vi "ROI Entry Screen.vi"() -> ()   [LabVIEW 2017]
uses:
  Typedefs/Line draw mode.ctl
  Typedefs/Top level VI states.ctl
  ROI Entry screen/Typedefs/ROI move buttons.ctl
  ROI Entry screen/Typedefs/ROI move mode.ctl
  Typedefs/Offsets cluster.ctl
  Typedefs/ROI management FG states.ctl
  ROI Entry screen/SubVIs/Automatic POI detection/Typedefs/Duplicate POI function enum.ctl
  ROI Entry screen/Typedefs/ROI entry screen ctrl refs cluster.ctl
  Typedefs/Read Write Enum.ctl
  Global Variables/General Globals.vi
  User profiles code/Globals/gl_UsrProfiles globals.vi
  ROI Entry screen/Globals/gl_ROI Entry UI globals.vi
  ROI Entry screen/Typedefs/ROI input mode.ctl
panel:
  out "Current ROI Type":string
  out "AOL Z ind. (um)":dbl caption="Motor Z" format="AOL Z   =  %#_g µm"
  out "# POI":i32 format="%.0f ROI"
  in  "Max Z Proj":bool
  out "ROI":T1
  out "Number of lines left":i32 format="%.0f number of lines left"
  in  "Palette Type":T2(ring)
  out "Zplane ind":i32 caption="Z-Plane" format="Z-Plane %.0f"
  in  "Z-Plane Selector":i32(c297)=7
  out "Image Display":T3(plugin-control)
  out "Motor Z ind. (um)":dbl caption="Motor Z" format="Motor Z = %#_g µm"
  out "# of planes":i32 format="# of Planes = %.0f"
  in  "Intensity slider":cluster{i16, i16}(slide)={0, 4095} caption="Intensity" scale=0.0..4095.0
  in  "Z-stack folder path":path caption="Experiment folder path"
  in  "Channel":enum16{"Green", "Red"}(ring)
  in  "Enable cool-down time":bool caption="Enable stimulus"
  in  "Cool-down time (s)":dbl caption="Cool-down time" min=0.0 max=60.0 step=0.05 format="%#.2f s"
  in  "Enable funct. stimulus":bool caption="Enable stimulus"
  in  "Funct stim.trig.delay (sec)":dbl=0.5 caption="Stimulus trigger delay" min=0.0 max=60.0 step=0.001 format="%#.3fs"
  in  "ROI move mode":T4
  in  "ROI offset arrows":T5
  in  "Trial Length (sec)":dbl=1.0 caption="Trial Length" min=0.05 max=60.0 step=1.0 format="%#.3f s"
  in  "Arb Plane Entry":bool caption="Load\nolder\nPOI"
  in  "Load ROI File":bool caption="Load\nolder\nPOI"
  in  "POI Density":dbl(slide) scale=0.01..1.0
  in  "Auto Generate":bool
  in  "Equal size":bool=TRUE
  in  "Whole plane":bool
  in  "Zoom":dbl=1.0 min=0.001 max=10.0 step=0.1 format="%#.2f x"
  out "Next State":T6=enum."Live Imaging-START"
  in  "Scan dwell time per pixel (us)":dbl=0.1 caption="Scan dwell time\nper pixel (us)" min=0.05 max=20.0 step=0.01 format="%.2f"
  in  "POI dwell time (us)":dbl=4.0 caption="POI dwell time" min=0.05 max=20.0 format="%_3g µs"
  in  "Live Imaging":bool
  in  "Acquisition":bool
  in  "Line Mode":T7=enum."Orthogonal"
  in  "Number of Trials":u16=1 min=1 max=1000 format="%.0f trials"
  in  "Wavelength (nm)":dbl=920.0 caption="Wavelength" min=800.0 max=1080.0 step=1.0 format="%#_g nm"
  in  "Done/Close":bool
  in  "Clear Last":bool
  in  "Clear All":bool
  in  "POISelect Array":cluster{"System Array":dbl[], "Boolean":bool}[](array[cluster])
  in  "Step size (µm)":u8(slide)=1 min=1 max=100 step=1 scale=1.0..30.0
  # "ROI Removal"
  # "ROI Input"
  # "ROI AutoGen"
  # "Min"
  # "Max"
  # "Stimulus trigger delay"
  # "Cool-down time"
  # "ROI Offset"
  # "Settings"
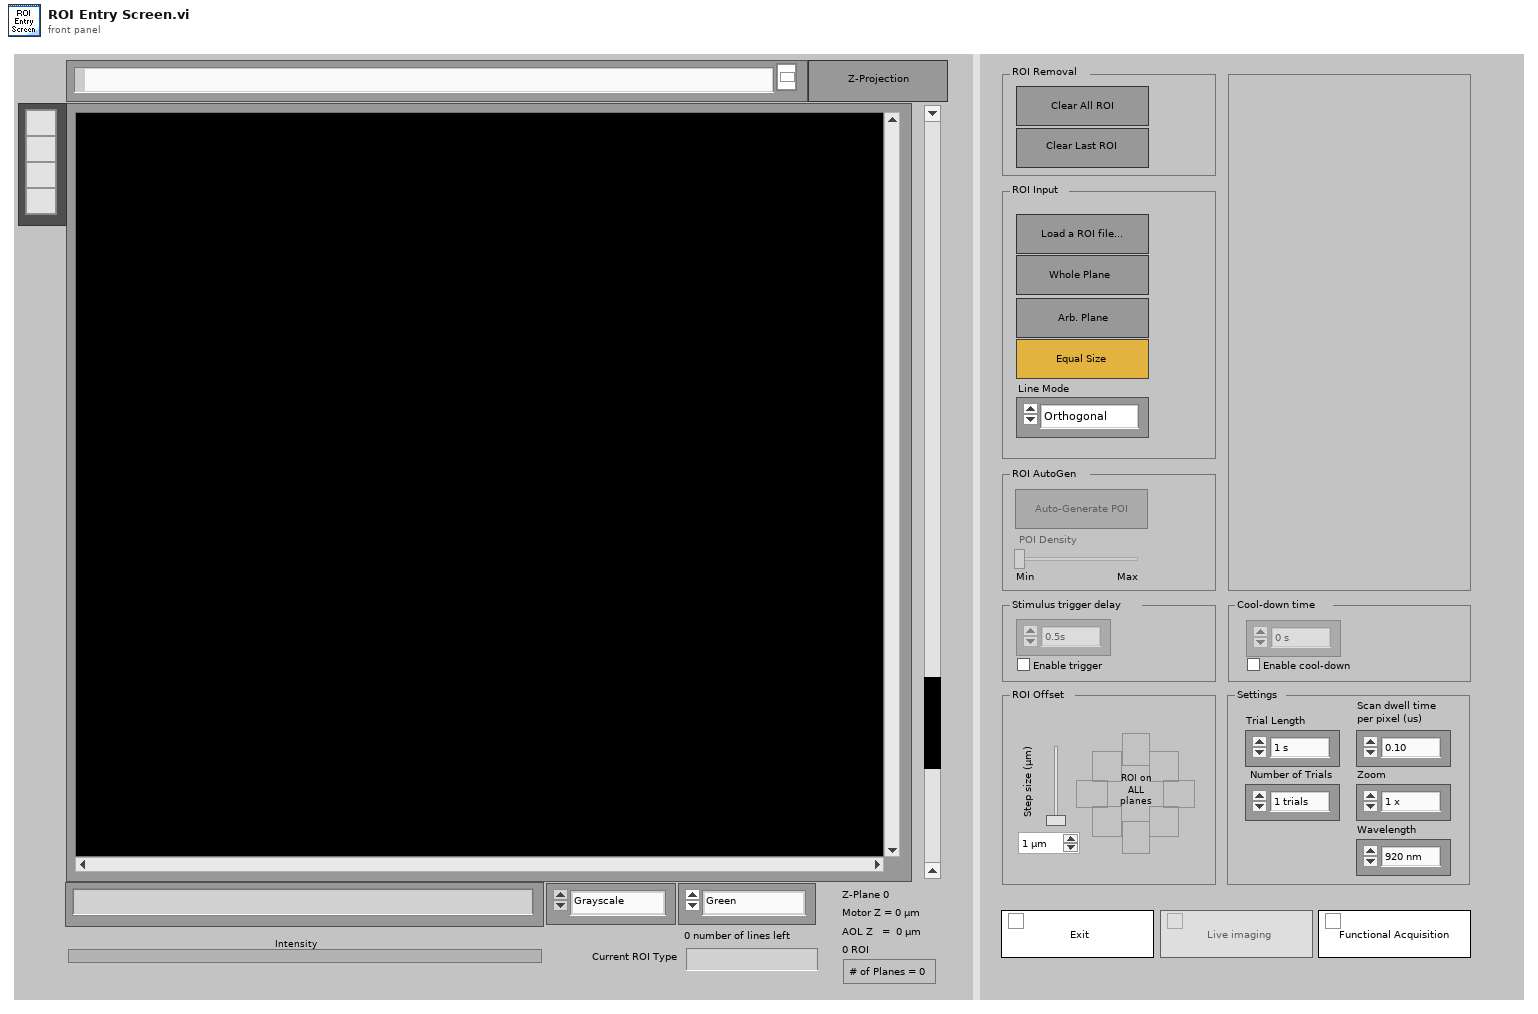
[diagram p1: front panel]
types:
  T1 = cluster{"Global Rectangle":i32[], "Contours":cluster{"Contour Type":u32, "ROI Type":u32, "Points":i32[]}[]}
  T2 = enum16{"Grayscale", "Binary", "Gradient", "Rainbow", "Temperature", "User Defined"}
  T3 = typedef "IMAQ Image.ctl" = refnum<image>
  T4 = typedef "ROI move mode.ctl" = enum16{"ROI on ALL planes", "ROI on current plane"}
  T5 = typedef "ROI move buttons.ctl" = cluster{"Right":bool, "Left":bool, "Up":bool, "Down":bool, "Up-left":bool, "Up-right":bool, "Down-left":bool, "Down-right":bool}
  T6 = typedef "Top level VI states.ctl" = enum16{"None", "Initialise UI", "<STACK PROTOCOL STATES>", "AOL Zstack-START", "AOL Zstack-STOP", "Motor Zstack-START", "Motor Zstack-STOP", "<ACQUISITION PROTOCOL STATES> ", "Functional Acquisition-START", "Functional Acquisition-STOP", "Single Plane Acquisition-START", "Single Plane Acquisition-STOP", "Volume Acquisition-START", "Volume Acquisition-STOP", "<LIVE IMAGING PROTOCOL STATES>", "Live Imaging-START", "Live Imaging-STOP", "Live Plane Imaging-START", "Live Plane Imaging-STOP", "Live Volume Imaging-START", "Live Volume Imaging-STOP", "<MOVEMENT CORRECTION PROTOCOL STATES>", "EXIT"}
  T7 = typedef "Line draw mode.ctl" = enum16{"Free draw", "Orthogonal"}
  T8 = typedef "Offsets cluster.ctl" = cluster{"X offset":i8, "Y offset":i8}
  T9 = cluster{"Load experiment data":refnum<user-event>, "Finish rectangle editing":refnum<user-event>, "Offset all ROI":refnum<user-event>}
  T10 = typedef "ROI info cluster.ctl" = cluster{"Global Rectangle":i32[], "Contours":cluster{"Contour Type":u32, "ROI Type":u32, "Points":i32[]}[]}
  T11 = typedef "ROI management FG states.ctl" = enum16{"Read", "Write", "Write-from dataset", "Clear Last", "Clear All", "Update ROIs time", "Reload last ROI set", "Offset all ROI", "Offset visible ROI"}
  T12 = typedef "ROI input mode.ctl" = enum16{"Unspecified", "Point-Line-Plane", "Volume"}
  T13 = enum8{"Enabled", "Disabled", "Disabled and Grayed Out"}
  T14 = typedef "Duplicate POI function enum.ctl" = enum16{"Generate", "Adjust number of POI", "Clear register"}
  T15 = typedef "ROI entry screen ctrl refs cluster.ctl" = cluster{"Done button":refnum<vi>, "Imaging button":refnum<vi>, "Acquisition button":refnum<vi>, "POI dwell time (us)":refnum<vi>, "Scan dwell time per pixel (us)":refnum<vi>, "# of planes":refnum<vi>, "Zoom Ctrl":refnum<vi>, "Equal size":refnum<vi>, "Channel":refnum<vi>, "Image Display":refnum<vi>, "Z-Plane Selector":refnum<vi>, "Number of lines left":refnum<vi>, "Z-stack folder path":refnum<vi>, "POI Density":refnum<vi>, "Arb Plane Entry":refnum<vi>, "Whole plane":refnum<vi>, "Clear Last":refnum<vi>, "Clear All":refnum<vi>, "Trial Length (sec)":refnum<vi>, "Palette Type":refnum<vi>, "Intensity slider":refnum<vi>, "# POI":refnum<vi>, "Max Z Proj":refnum<vi>, "Zplane ind":refnum<vi>, "Wavelength (nm)":refnum<vi>, "Number of Trials":refnum<vi>, "Funct stim.trig.enable":refnum<vi>, "Funct stim.trig.delay (s)":refnum<vi>, "Line Mode":refnum<vi>, "Step size (µm)":refnum<vi>, "ROI move mode":refnum<vi>, "Cool-down time (s)":refnum<vi>, "Enable cool-down time":refnum<vi>, "Motor Z ind. (um)":refnum<vi>, "AOL Z ind. (um)":refnum<vi>}
  T16 = typedef "Read Write Enum.ctl" = enum16{"Read", "Write"}
  T17 = typedef "ROI ID Enum.ctl" = enum16{"Point", "MiniScan", "Comp. MiniScan", "Rectangle", "Comp. volume", "Arb. plane point", "None"}
  T18 = typedef "lveventtype.ctl" = enum32{"Null", "Timeout", "Annotation Menu Selection", "Annotation Menu Selection?", "App Instance Close", "App Instance Close?", "Autoscale Range Change", "Bookmark Info Change", "Cell Edit", "Cell Edit?", "Cursor Grab", "Cursor Grab?", "Cursor Menu Selection", "Cursor Menu Selection?", "Cursor Move", "Cursor Release", "Data Change", "Direction Change", "Display State Change", "Drag Ended", "Drag Enter", "Drag Leave", "Drag Over", "Drag Source Update", "Drag Starting", "Drag Starting?", "Drop", "Exec State Change", "Key Down", "Key Down?", "Key Repeat", "Key Repeat?", "Key Up", "Listbox Double Click", "Menu Activation?", "Menu Selection (App)", "Menu Selection? (App)", "Menu Selection (User)", "Mouse Down", "Mouse Down?", "Mouse Enter", "Mouse Leave", "Mouse Move", "Mouse Up", "Mouse Wheel", "NI Security User Change (App)", "Pane Size", "Panel Close", "Panel Close?", "Panel Resize", "Plot Attribute Change", "Scale Range Change", "Shortcut Menu Activation?", "Shortcut Menu Selection (App)", "Shortcut Menu Selection? (App)", "Shortcut Menu Selection (User)", "Tree Double Click", "Tree Drag", "Tree Drag?", "Tree Drop", "Tree Drop?", "Tree Item Close", "Tree Item Close?", "Tree Item Open", "Tree Item Open?", "User Event", "Value Change"}
  T19 = typedef "ROI Entry screen VI interface 1.ctl" = cluster{"Last Image Display Event info":T20, "ROIs Info []":T21[], "Cancelled":bool, "Done button disabled?":enum8{"Enabled", "Disabled", "Disabled and Grayed Out"}, "Acquisition button disabled?":enum8{"Enabled", "Disabled", "Disabled and Grayed Out"}}
  T20 = typedef "Last Image Display Event info.ctl" = cluster{"Type":i32, "Tool":i32, "Coordinates":i32[], "Other Parameters":sgl[]}
  T21 = typedef "ROI spec.ctl" = cluster{"Coordinates":i32[], "Zoom":dbl, "ROI Enum":T17, "Z planeIdx(s)":i32[], "Z planecodes(s)":u8[], "Z start":dbl, "Z stop":dbl}
  T22 = typedef "ROI parameters data type.ctl" = cluster{"ROI index":dbl, "ROI ID":dbl, "ROI Time (ns)":dbl, "Pixels in ROI":dbl, "X start":dbl, "Y start":dbl, "Z start":dbl, "X stop":dbl, "Y stop":dbl, "Z stop":dbl, "Angle (deg)":dbl, "Composite ID":dbl, "Number of lines":dbl, "Frame Size":dbl, "Zoom":dbl, "Laser Power (%)":dbl, "ROI group ID":dbl, "Z Plane Idx":i32[], "Z Plane codes":i32[]}
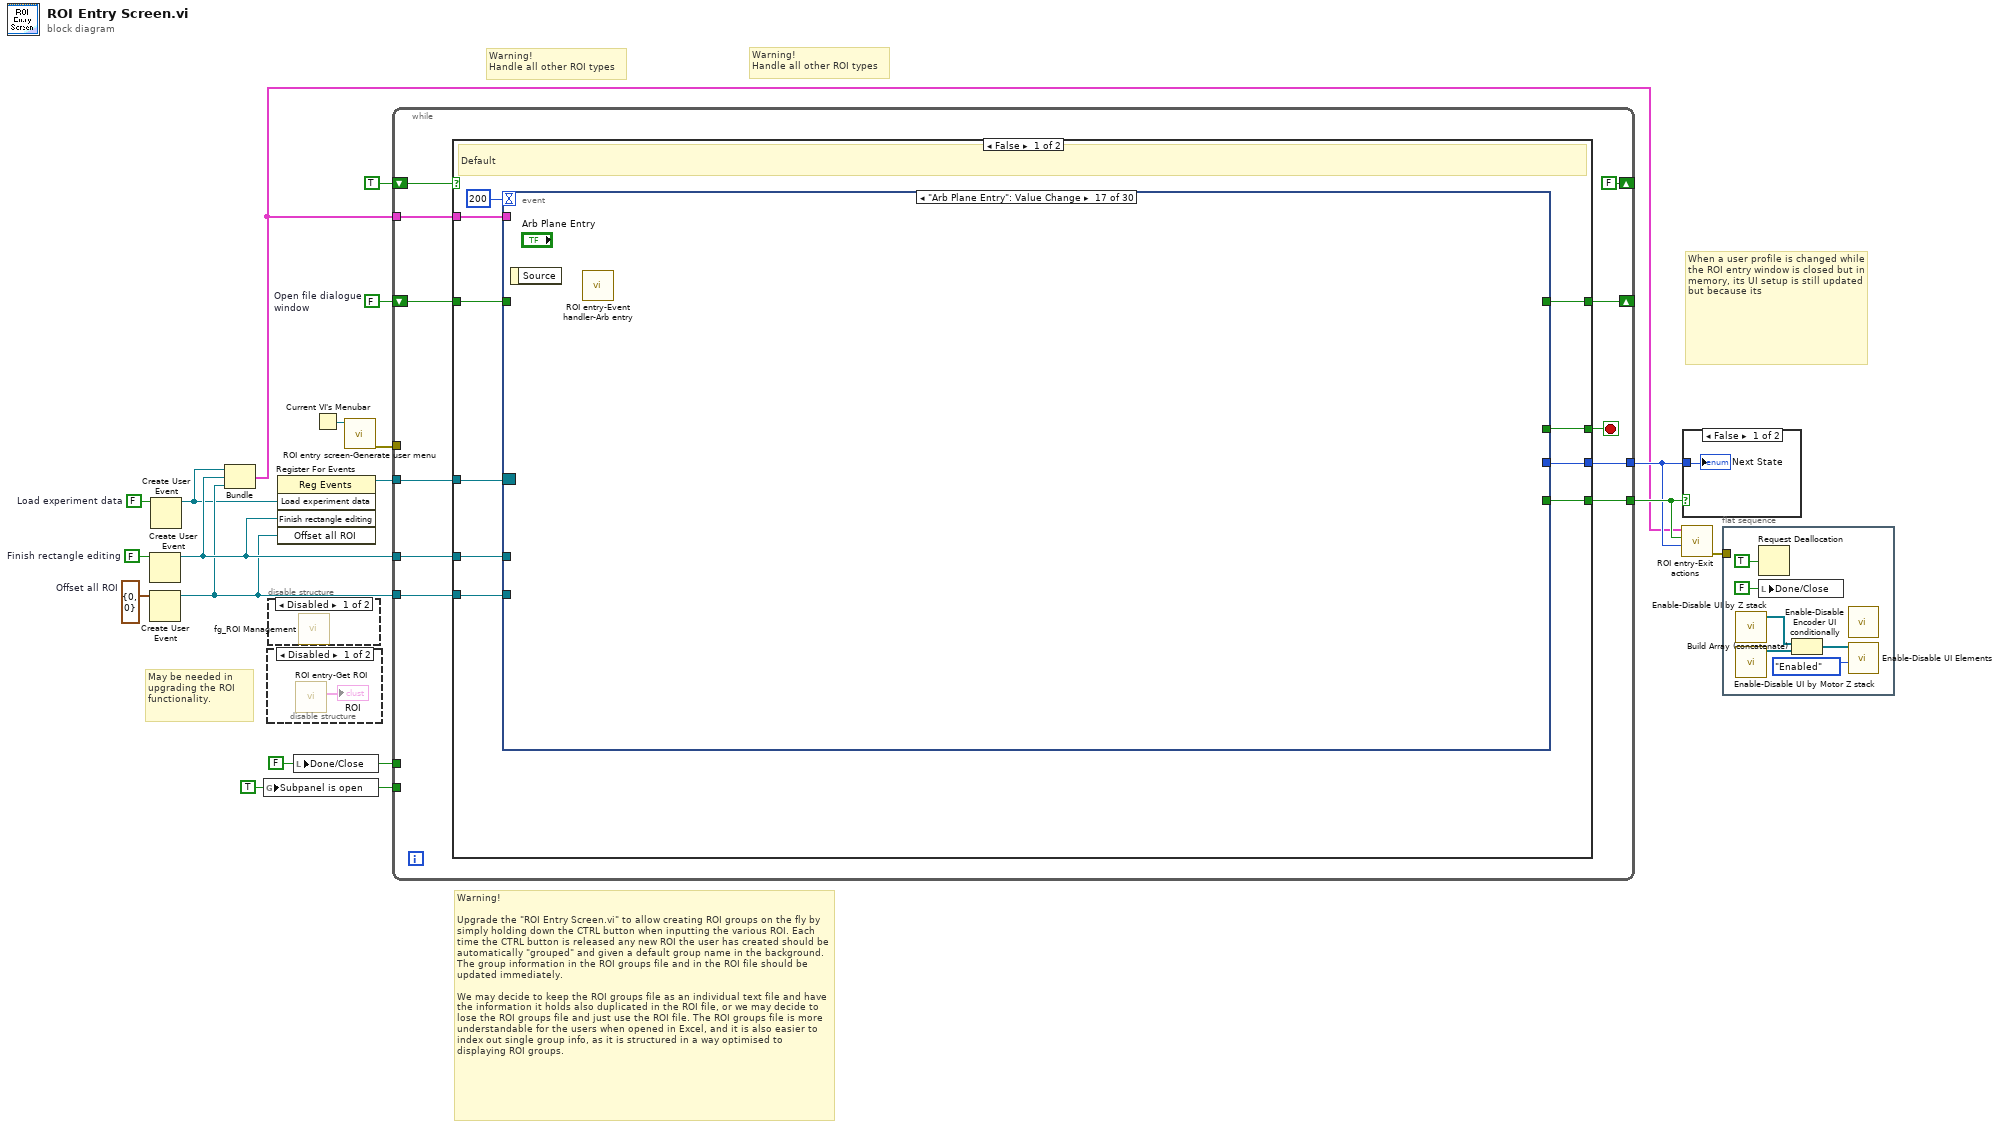
[diagram p0: block diagram]
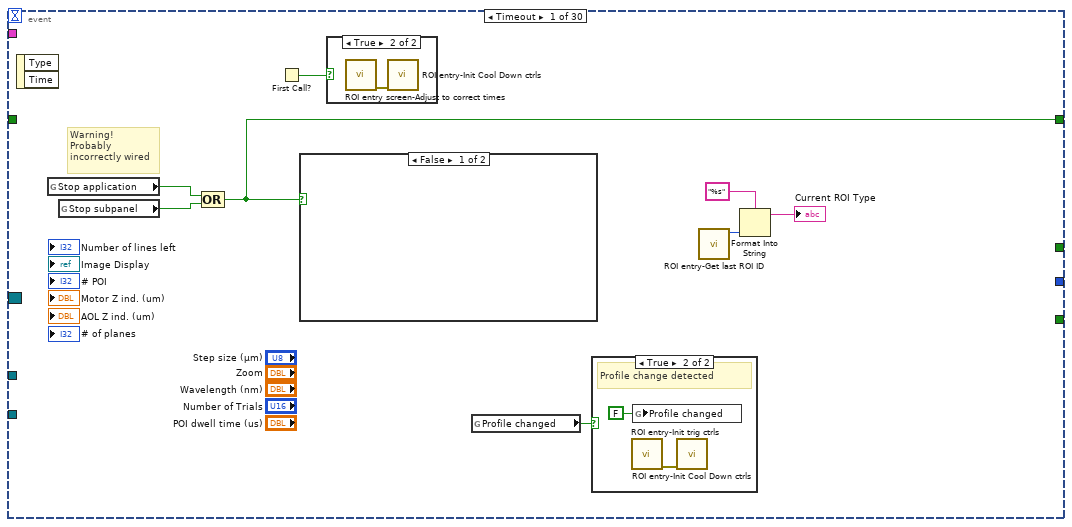
[diagram p5: hidden frame]
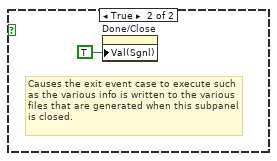
[diagram p8: hidden frame]
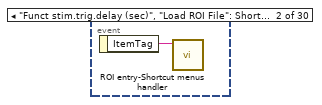
[diagram p9: hidden frame]
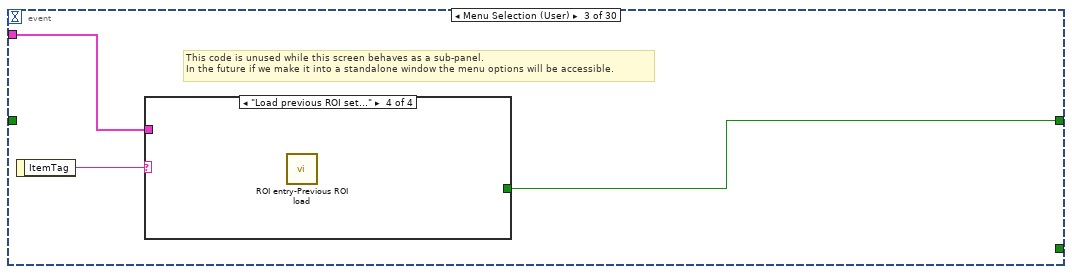
[diagram p10: hidden frame]
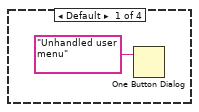
[diagram p11: hidden frame]
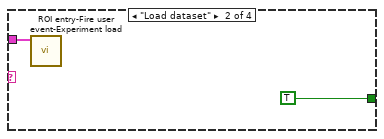
[diagram p12: hidden frame]
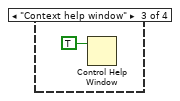
[diagram p13: hidden frame]
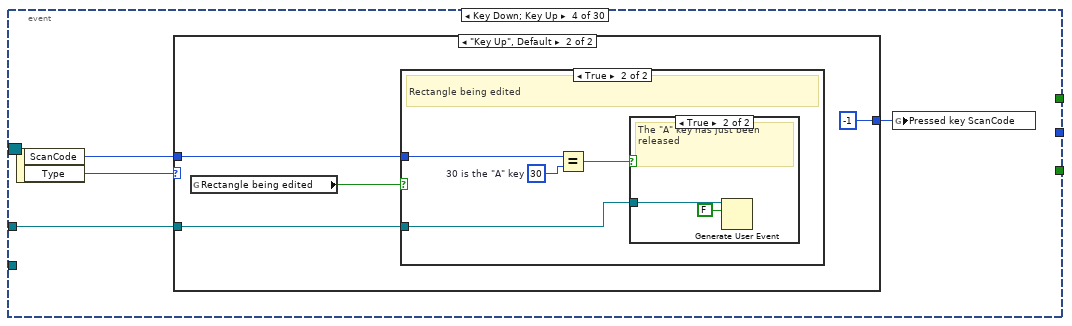
[diagram p14: hidden frame]
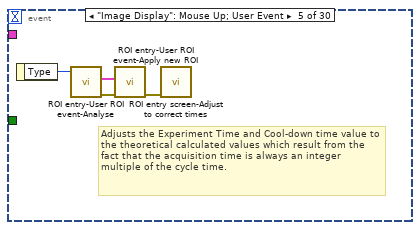
[diagram p18: hidden frame]
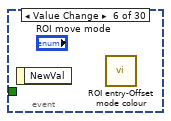
[diagram p19: hidden frame]
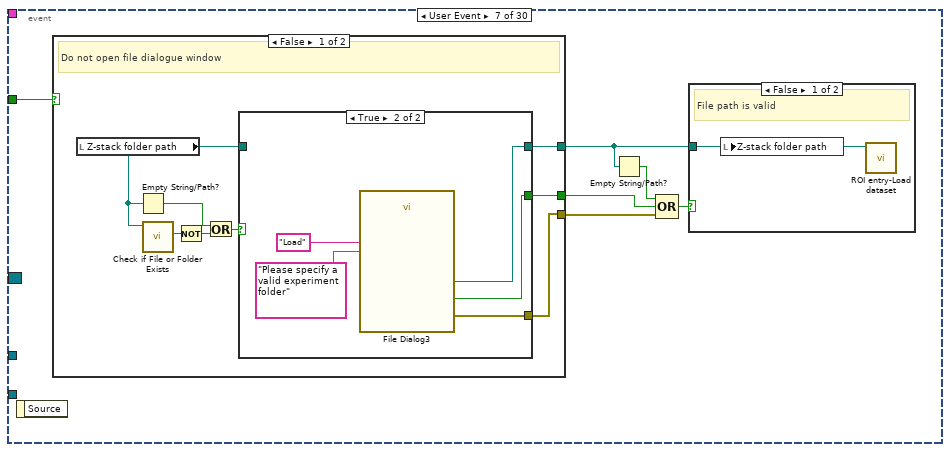
[diagram p20: hidden frame]
diagram:
  w5 = T8 {"X offset"=0, "Y offset"=0}  # Offset all ROI
  w6 = FALSE ("Done/Close")
  w12 = FALSE  # Finish rectangle editing
  w14 = TRUE ("Subpanel is open")
  w15 = FALSE  # Open file dialogue window
  w17 = FALSE  # Load experiment data
  # "When a user profile is changed while the ROI entry window is closed but in memory, its UI setup is still updated but because its"
  # "Warning!\n\nUpgrade the \"ROI Entry Screen.vi\" to allow creating ROI groups on the fly by simply holding down the CTRL button when inputting the various ROI. Each time the CTRL button is released any new ROI the user has created should be automatically \"grouped\" and given a default group name in the background. The group information in the ROI groups file and in the ROI file should be updated immediately.\n\nWe may decide to keep the ROI groups file as an individual text file and have the information it holds also duplicated in the ROI file, or we may decide to lose the ROI groups file and just use the ROI file. The ROI groups file is more understandable for the users when opened in Excel, and it is also easier to index out single group info, as it is structured in a way optimised to displaying ROI groups."
  # "May be needed in upgrading the ROI functionality."
  # "Warning!\nHandle all other ROI types"
  # "Warning!\nHandle all other ROI types"
  n1 = Create User Event(user event datatype=w12) -> (user event=w4:refnum<user-event>)  [unwired: 1 in, 1 out]
  n2 = Create User Event(user event datatype=w5) -> (user event=w3:refnum<user-event>)  [unwired: 1 in, 1 out]
  n3 = Create User Event(user event datatype=w17) -> (user event=w2:refnum<user-event>)  [unwired: 1 in, 1 out]
  n4 = Bundle("Load experiment data"=w2, "Finish rectangle editing"=w4, "Offset all ROI"=w3) -> (w1:T9)  [unwired: 1 in]
  n5 = global write "General Globals.vi" "Subpanel is open"(w14) -> ()
  n6 = disable-structure shown="Disabled" {
    frame Disabled {
      n7 = call "ROI entry-Get ROI.vi"() -> ("ROI info cluster (native format)"=→"ROI":T10)  [unwired: 10 in, 1 out]
    }
    frame Enabled {
    }
  }
  n8 = disable-structure shown="Disabled" {
    frame Disabled {
      n9 = call "fg_ROI Management.vi"() -> ()  [unwired: 6 in, 6 out]
    }
    frame Enabled {
    }
  }
  n10 = register-events(w2, w4, w3) -> (reference out=w16:refnum<event-registration>)  [unwired: 2 in, 1 out]
  n11 = local write "Done/Close"(w6) -> ()
  n12 = Current VI's Menubar() -> (w11:refnum<k9>)
  n13 = call "ROI entry screen-Generate user menu.vi"("Functional Viewer Menu in"=w11) -> ("error out"=w10:errorcluster)  [unwired: 9 in, 1 out]
  n14 = while {
    shift-right: [FALSE] -> _
    shift-left: TRUE -> [w28]
    tunnel: [w26] -> w8
    tunnel: w16 -> [w25]
    tunnel: w1 -> [w24]
    shift-right: [w23] -> _
    shift-left: w15 -> [w22]
    tunnel: w14 -> [_]
    tunnel: w4 -> [w21]
    tunnel: w10 -> [_]
    tunnel: [w20] -> w9
    tunnel: w6 -> [_]
    tunnel: w3 -> [w19]
    stop <- w29 stop-if-true
    n15 = case shown="False" w28 {
      tunnel: [w38 _] -> w29
      tunnel: [w37 _] -> w26
      tunnel: w25 -> [w36 _]
      tunnel: w24 -> [w35 w267]
      tunnel: [w33 w268] -> w23
      tunnel: w22 -> [w34 _]
      tunnel: w21 -> [w32 _]
      tunnel: [w31 _] -> w20
      tunnel: w19 -> [w30 _]
      frame False {
        # "Default"
        n16 = event shown="[16] \"Arb Plane Entry\": Value Change" {
          selector: w36 -> [_ _ _ _ _ _ _ _ _ _ _ _ _ _ _ _ _ _ _ _ _ _ _ _ _ _ _ _ _ _]
          dyn-events: _ -> [_ _ _ _ _ _ _ _ _ _ _ _ _ _ _ _ _ _ _ _ _ _ _ _ _ _ _ _ _ _]
          timeout: 200 -> [_ _ _ _ _ _ _ _ _ _ _ _ _ _ _ _ _ _ _ _ _ _ _ _ _ _ _ _ _ _]
          tunnel: [_ _ _ _ _ _ _ _ _ _ _ _ _ _ _ _ _ _ _ _ _ _ _ _ w256 _ _ _ _ w265] -> w38
          tunnel: [_ _ _ _ _ _ _ _ _ _ _ _ _ _ _ _ _ _ _ _ _ _ _ _ w257 _ _ _ _ _] -> w37
          tunnel: w35 -> [_ _ w54 _ _ _ _ _ _ _ _ w161 _ _ _ _ _ _ _ _ _ _ _ _ _ _ _ _ _ _]
          tunnel: w34 -> [_ _ _ _ _ _ w83 _ _ w157 _ _ _ _ _ _ _ _ _ _ _ _ _ _ _ _ _ _ _ _]
          tunnel: [w46 _ w53 _ _ _ _ _ _ _ _ _ _ _ _ _ _ _ _ _ _ _ _ _ _ _ _ _ _ _] -> w33
          tunnel: w32 -> [_ _ _ w63 _ _ _ _ _ _ _ _ _ _ _ _ _ _ _ _ _ _ _ _ _ _ _ _ _ _]
          tunnel: [_ _ _ _ _ _ _ _ _ _ _ _ _ _ _ _ _ _ _ _ _ _ _ _ _ _ _ _ _ w265] -> w31
          tunnel: w30 -> [_ _ _ _ _ _ _ _ w156 _ _ _ _ _ _ _ _ _ _ _ _ _ _ _ _ _ _ _ _ _]
          event Timeout {
            # "Warning!\nProbably\nincorrectly wired"
            n17 = event-data() -> ()  [unwired: 1 in, 2 out]
            n18 = global read "General Globals.vi" "Stop application"() -> (w47:bool)
            n19 = global read "General Globals.vi" "Stop subpanel"() -> (w45:bool)
            n20 = Compound Arithmetic op=OR(w47, w45) -> (w46:bool)
            n21 = First Call?() -> (First Call?: T/F=w40:bool)
            n22 = case shown="False" w46 {
              frame False {
              }
              frame True {
                # "Causes the exit event case to execute such as the various info is written to the various files that are generated when this subpanel is closed."
                n23 = property on="Done/Close" class="Bool (strict)"("Val(Sgnl)"=TRUE) -> ()  [unwired: 2 in, 2 out]
              }
            }
            n24 = case shown="True" w40 {
              frame False {
              }
              frame True {
                n25 = call "ROI entry screen-Adjust to correct times.vi"() -> ("error out"=w50:errorcluster)  [unwired: 10 in, 1 out]
                n26 = call "ROI entry-Init Cool Down ctrls.vi"("error in (no error)"=w50) -> ()  [unwired: 10 in, 1 out]
              }
            }
            n27 = global read "gl_UsrProfiles globals.vi" "Profile changed"() -> (w44:bool)
            n28 = case shown="True" w44 {
              frame False {
                # "Idle"
              }
              frame True {
                # "Profile change detected"
                n29 = call "ROI entry-Init trig ctrls.vi"() -> ("error out"=w49:errorcluster)  [unwired: 11 in]
                n30 = global write "gl_UsrProfiles globals.vi" "Profile changed"(FALSE ("Profile changed")) -> ()
                n31 = call "ROI entry-Init Cool Down ctrls.vi"("error in (no error)"=w49) -> ()  [unwired: 10 in, 1 out]
              }
            }
            n32 = call "ROI entry-Get last ROI ID.vi"() -> ("ROI ID Enum"=w43:T17)  [unwired: 8 in, 3 out]
            n33 = Format Into String(format string="%s", w43) -> (resulting string=→"Current ROI Type":string)  [unwired: 2 in, 1 out]
          }
          event "Funct stim.trig.delay (sec)", "Load ROI File": Shortcut Menu Selection (User) {
            n34 = event-data() -> ("ItemTag"=w52:string)  [unwired: 1 in]
            n35 = call "ROI entry-Shortcut menus handler.vi"("ItemTag"=w52) -> ()  [unwired: 11 in]
          }
          event Menu Selection (User) {
            # "This code is unused while this screen behaves as a sub-panel.\nIn the future if we make it into a standalone window the menu options will be accessible."
            n36 = event-data() -> ("ItemTag"=w55:string)  [unwired: 1 in]
            n37 = case shown="\"Load previous ROI set...\"" w55 {
              tunnel: w54 -> [_ w57 _ _]
              tunnel: [_ TRUE _ _] -> w53
              frame Default {
                n38 = One Button Dialog(message="Unhandled user menu") -> ()  [unwired: 1 in, 1 out]
              }
              frame "Load dataset" {
                n39 = call "ROI entry-Fire user event-Experiment load.vi"("User Events Cluster"=w57) -> ()  [unwired: 10 in, 1 out]
              }
              frame "Context help window" {
                n40 = Control Help Window(1:TRUE ("Show")) -> ()  [unwired: 1 in]
              }
              frame "Load previous ROI set..." {
                n41 = call "ROI entry-Previous ROI load.vi"() -> ()  [unwired: 11 in, 1 out]
              }
            }
          }
          event Key Down; Key Up {
            n42 = event-data() -> ("ScanCode"=w62:i16, "Type"=w61:T18)  [unwired: 1 in]
            n43 = case shown="\"Key Up\", Default" w61 {
              tunnel: w63 -> [_ w68]
              tunnel: w62 -> [w64 w67]
              tunnel: [w64 i16 -1 ("ScanCode")] -> w60
              frame "Key Down" {
              }
              frame "Key Up", Default {
                n44 = global read "gl_ROI Entry UI globals.vi" "Rectangle being edited"() -> (w66:bool)
                n45 = case shown="True" w66 {
                  tunnel: w67 -> [_ w71]
                  tunnel: w68 -> [_ w70]
                  frame False {
                  }
                  frame True {
                    w72 = i16 30  # 30 is the "A" key
                    # "Rectangle being edited"
                    n46 = Equal?(x=w71, y=w72) -> (x = y?=w69:bool)
                    n47 = case shown="True" w69 {
                      tunnel: w70 -> [_ w74]
                      frame False {
                      }
                      frame True {
                        # "The \"A\" key has just been released"
                        n48 = Generate User Event(user event=w74, event data cluster=FALSE ("event data")) -> ()  [unwired: 2 in, 2 out]
                      }
                    }
                  }
                }
              }
            }
            n49 = global write "gl_ROI Entry UI globals.vi" "Pressed key ScanCode"(w60) -> ()
          }
          event "Image Display": Mouse Up; User Event {
            # "Adjusts the Experiment Time and Cool-down time value to the theoretical calculated values which result from the fact that the acquisition time is always an integer multiple of the cycle time."
            n50 = event-data() -> ("Type"=w78:u32)  [unwired: 1 in]
            n51 = call "ROI entry-User ROI event-Analyse.vi"("Event Type"=w78) -> ("error out"=w76:errorcluster, "output cluster"=w77:T19)  [unwired: 9 in]
            n52 = call "ROI entry-User ROI event-Apply new ROI.vi"("error in (no error)"=w76, "Input cluster"=w77) -> ("error IO"=w75:errorcluster)  [unwired: 9 in]
            n53 = call "ROI entry screen-Adjust to correct times.vi"("error in (no error)"=w75) -> ()  [unwired: 9 in, 2 out]
          }
          event Value Change {
            n54 = event-data() -> ()  [unwired: 1 in, 1 out]
            n55 = call "ROI entry-Offset mode colour.vi"() -> ()  [unwired: 11 in, 1 out]
          }
          event User Event {
            n56 = event-data() -> ()  [unwired: 1 in, 1 out]
            n57 = case shown="False" w83 {
              tunnel: [w87 w102] -> w84
              tunnel: [w85 w101] -> w82
              tunnel: [w86 w100] -> w81
              frame False {
                # "Do not open file dialogue window"
                n58 = local read "Z-stack folder path"() -> (w88:path)
                n59 = Empty String/Path?(string/path=w88) -> (empty?=w92:bool)
                n60 = call <vilib>:"Check if File or Folder Exists.vi"("path"=w88) -> ("file or folder exists?"=w90:bool)  [unwired: 8 in, 2 out]
                n61 = Not(x=w90) -> (.not. x?=w91:bool)
                n62 = Or(x=w92, y=w91) -> (x .or. y?=w89:bool)
                n63 = case shown="True" w89 {
                  tunnel: w88 -> [w93 _]
                  tunnel: [w93 w97] -> w87
                  tunnel: [_ w96] -> w86
                  tunnel: [_ w95] -> w85
                  frame False {
                  }
                  frame True {
                    n64 = call "File Dialog3"("prompt"="Please specify a valid experiment folder", "button label"="Load") -> ("selected path"=w97:path, "cancelled"=w95:bool, "error out"=w96:errorcluster)  [unwired: 10 in, 1 out]
                  }
                }
              }
              frame True {
                # "Open file dialogue window"
                n65 = call "File Dialog2"("prompt"="Please specify a valid experiment folder", "button label"="Load") -> ("selected path"=w102:path, "cancelled"=w101:bool, "error out"=w100:errorcluster)  [unwired: 10 in, 1 out]
              }
            }
            n66 = Empty String/Path?(string/path=w84) -> (empty?=w80:bool)
            n67 = Compound Arithmetic op=OR(w80, w82, w81) -> (w79:bool)
            n68 = case shown="False" w79 {
              tunnel: w84 -> [w104 _]
              frame False {
                # "File path is valid"
                n69 = local write "Z-stack folder path"(w104) -> ()
                n70 = call "ROI entry-Load dataset.vi"("Experiment folder path OR Z-stack folder path"=w104) -> ()  [unwired: 10 in, 1 out]
              }
              frame True {
                # "Empty file path / Not a path / User cancelled / Error"
              }
            }
          }
          event User Event {
            n71 = event-data() -> ("X offset"=w106:i8, "Y offset"=w105:i8)  [unwired: 1 in]
            n72 = disable-structure shown="Disabled" {
              disable-tunnel: w106 -> [_ w154]
              disable-tunnel: w105 -> [_ w153]
              frame Disabled {
                w107 = 0.0  # Y Offset
                w108 = 0.0  # X Offset
                # "WARNING!\nOld functionality.\nMust be upgraded for rig 3."
                n73 = call "POISelection.vi"("POISelectArrayIn"="POISelect Array") -> ("POI array"=w124:dbl[][])  [unwired: 9 in, 1 out]
                n74 = Index Array(array=w124, index (col) #1=1 ("index (row)"), index (col) #2=2 ("index (col)")) -> (element #1=w125:dbl[], element #2=w117:dbl[])  [unwired: 2 in]
                n75 = Add(x=w125, y=w108) -> (x+y=w123:dbl[])
                n76 = Add(x=w117, y=w107) -> (x+y=w116:dbl[])
                n77 = Replace Array Subset(array=w124, new element #1=w123, index (col) #1=1 ("disabled index (col)"), new element #2=w116, index (col) #2=2 ("index (col)")) -> (w119:dbl[][])  [unwired: 2 in]
                n78 = call "ROI entry-Get selected Z-plane index.vi"() -> ("Z-plane selector (index)"=w109:i32)  [unwired: 10 in, 1 out]
                n79 = call "ROI entry-Get Max Proj setting.vi"() -> ("Max Z-projection setting's value"=w110:bool)  [unwired: 10 in, 1 out]
                n80 = call "ROI entry-Clear ROI overlay.vi"() -> ("error out"=w112:errorcluster, "Image Out"=w113:T3)  [unwired: 10 in]
                n81 = for {
                  tunnel: w119 -> [w132] mode=indexing
                  shift-right: [w135] -> w111
                  shift-left: w113 -> [w134]
                  tunnel: w109 -> [w128]
                  tunnel: w112 -> [_]
                  tunnel: w110 -> [w126]
                  n82 = Index Array(array=w132, index=3) -> (element=w130:dbl)
                  n83 = Delete From Array(array=w132, index=0) -> (deleted portion=w127:dbl, array with subset deleted=w133:dbl[])  [unwired: 1 in]
                  n84 = Equal?(x=w130, y=w128) -> (x = y?=w129:bool)
                  n85 = case shown="True" w126 {
                    tunnel: [w141 w152] -> w135
                    tunnel: w134 -> [w140 w151]
                    tunnel: w133 -> [w139 w150]
                    tunnel: w129 -> [w138 _]
                    tunnel: w127 -> [w137 w149]
                    frame False {
                      n86 = case shown="True" w138 {
                        tunnel: [w142 w147] -> w141
                        tunnel: w140 -> [w142 w146]
                        tunnel: w137 -> [_ w145]
                        tunnel: w139 -> [_ w143]
                        frame False {
                        }
                        frame True {
                          n87 = Increment(x=w145) -> (x+1=w144:dbl)
                          n88 = call "PointOverlayV1.vi"("Point"=w143, "Count"=w144, "Image1"=w146) -> ("Image1 Out"=w147:T3)  [unwired: 8 in]
                        }
                      }
                    }
                    frame True {
                      n89 = Increment(x=w149) -> (x+1=w148:dbl)
                      n90 = call "PointOverlayV1.vi"("Point"=w150, "Count"=w148, "Image1"=w151) -> ("Image1 Out"=w152:T3)  [unwired: 8 in]
                    }
                  }
                }
                n91 = call "POIConvert.vi"("POI array"=w119) -> ("POISelectArrayOut"=w122:cluster{"System Array":dbl[], "Boolean":bool}[])  [unwired: 10 in]
                n92 = local write "POISelect Array"(w122) -> ()
                n93 = call "ROI entry-Image display write.vi"("Value"=w111) -> ()  [unwired: 4 in, 1 out]
              }
              frame Enabled {
                n94 = call "ROI entry-Offset all ROI.vi"("Y offset"=w153, "X offset"=w154) -> ()  [unwired: 9 in, 1 out]
              }
            }
          }
          event Value Change {
            n95 = event-data() -> ("NewVal"=w155:T5)  [unwired: 1 in]
            n96 = call "ROI entry-Event handler-ROI offset.vi"("Offset all ROI-User Event in"=w156, "ROI offset arrows: NewVal"=w155) -> ()  [unwired: 9 in, 1 out]
          }
          event "Load ROI File": Value Change {
            # "Adjusts the Experiment Time and Cool-down time value to the theoretical calculated values which result from the fact that the acquisition time is always an integer multiple of the cycle time."
            n97 = event-data() -> ()  [unwired: 1 in, 1 out]
            n98 = flat-sequence {
              tunnel: [w159] -> w158
              tunnel: w157 -> [_]
              tunnel: w158 -> [_]
              frame #0 {
                n99 = call "ROI entry-Previous ROI load.vi"() -> ("Proceed"=w159:bool)  [unwired: 11 in]
              }
              frame #1 {
                n100 = call "ROI entry screen-Adjust to correct times.vi"() -> ()  [unwired: 10 in, 2 out]
              }
            }
          }
          event Value Change {
            n101 = event-data() -> ()  [unwired: 1 in, 1 out]
            n102 = call "fgv_ROI equal size line coords.vi"("Function"=enum16{"Intialize", "Write", "Read", "Clear"}."Clear") -> ()  [unwired: 9 in, 2 out]
          }
          event "Z-stack folder path": Value Change {
            n103 = event-data() -> ()  [unwired: 1 in, 1 out]
            n104 = call "ROI entry-Fire user event-Experiment load.vi"("User Events Cluster"=w161) -> ()  [unwired: 10 in, 1 out]
          }
          event "Z-Plane Selector": Value Change {
            w164 = FALSE ("Max Z Proj")
            # "Max Z-projection button automatically released when the scrollbar is moved."
            # "Compensates for Labview bug."
            n105 = event-data() -> ()  [unwired: 1 in, 1 out]
            n106 = property on="Z-Plane Selector" class="Scroll (strict)"() -> ("DocMax"=w170:dbl, "DocMin"=w169:dbl)  [unwired: 2 in, 2 out]
            n107 = feedback-in #1("Z-Plane Selector") -> ()
            n108 = feedback #1() -> (w171:i32)  [unwired: 1 in]
            n109 = Decrement(x=w170) -> (x-1=w165:dbl)
            n110 = property on="Z-Plane Selector" class="Scroll (strict)"() -> ("PageSize"=w163:dbl)  [unwired: 2 in, 2 out]
            n111 = local write "Max Z Proj"(w164) -> ()
            n112 = Less?(x="Z-Plane Selector", y=w169) -> (x < y?=w168:bool)
            n113 = Greater?(x="Z-Plane Selector", y=w165) -> (0:w167:bool)
            n114 = feedback #2() -> (w162:dbl)  [unwired: 1 in]
            n115 = feedback-in #2(w163) -> ()
            n116 = Or(x=w167, y=w168) -> (x .or. y?=w166:bool)
            n117 = case shown="False" w166 {
              tunnel: w171 -> [_ w177]
              tunnel: "Z-Plane Selector" -> [w173 _]
              tunnel: w164 -> [_ _]
              tunnel: w162 -> [_ w178]
              frame False {
                # "Input value is in range"
                n118 = flat-sequence {
                  tunnel: w173 -> [w174]
                  frame #0 {
                    "Zplane ind" <- w174
                  }
                  frame #1 {
                    n119 = call "ROI entry-Handle ROI change.vi"("ROI management"=ROI_management_FG_states."Read") -> ("error out"=w175:errorcluster)  [unwired: 8 in, 2 out]
                    n120 = call "ROI entry-Index Zplane position.vi"("error in (no error)"=w175) -> ()  [unwired: 9 in, 2 out]
                  }
                }
              }
              frame True {
                # "Prevents out of range inputs"
                n121 = property on="Z-Plane Selector" class="Scroll (strict)"("PageSize"=w178) -> ()  [unwired: 2 in, 2 out]
                n122 = call "ROI entry-Set Z-plane selector.vi"("Z-plane selector value"=w177) -> ()  [unwired: 10 in, 1 out]
              }
            }
          }
          event "Channel", "Max Z Proj": Value Change {
            n123 = event-data() -> ()  [unwired: 1 in, 1 out]
            n124 = call "ROI entry-Event handler-Max projection.vi"() -> ()  [unwired: 11 in, 1 out]
          }
          event "Intensity slider": Value Change {
            n125 = event-data() -> ()  [unwired: 1 in, 1 out]
            n126 = call "ROI entry-Set display mapping.vi"() -> ()  [unwired: 11 in, 1 out]
          }
          event "Palette Type": Value Change {
            n127 = event-data() -> ("NewVal"=w179:T2)  [unwired: 1 in]
            n128 = call "ROI entry-Set palette type.vi"("Palette:Palette Type"=w179) -> ()  [unwired: 10 in, 1 out]
          }
          event "Arb Plane Entry": Value Change {
            n129 = event-data() -> ()  [unwired: 1 in, 1 out]
            n130 = call "ROI entry-Event handler-Arb entry.vi"() -> ()  [unwired: 11 in, 1 out]
          }
          event "Whole plane": Value Change {
            n131 = event-data() -> ()  [unwired: 1 in, 1 out]
            n132 = call "ROI entry-Event handler-Whole plane.vi"() -> ()  [unwired: 12 in]
          }
          event "Equal size": Value Change {
            n133 = event-data() -> ()  [unwired: 1 in, 1 out]
            n134 = call "ROI entry-Event handler-Equal Size.vi"() -> ()  [unwired: 12 in]
          }
          event "Auto Generate": Value Change {
            n135 = event-data() -> ()  [unwired: 1 in, 1 out]
            n136 = disable-structure shown="Disabled" {
              frame Disabled {
                n137 = call "fg_ROI Management.vi"("Function"=ROI_management_FG_states."Read") -> ("ROI Setup"=w183:T22[])  [unwired: 5 in, 5 out]
                n138 = Empty Array?(array=w183) -> (empty?=w182:bool)
                n139 = case shown="False" w182 {
                  tunnel: [w202 w205] -> w181
                  frame False {
                    # "User-specified ROIs exist"
                    n140 = Two Button Dialog(message="WARNING\n\nThe Auto-generate function will overwrite existing ROIs.\n", 2:"Proceed..." ("T button name (\"OK\")")) -> (T button?=w202:bool)  [unwired: 1 in]
                  }
                  frame True {
                    w205 = TRUE  # Proceed
                    # "No user-specified ROIs"
                  }
                }
                n141 = case shown="True" w181 {
                  frame False {
                  }
                  frame True {
                    n142 = call "POI Autogen number entry window.vi"() -> ("Cancelled"=w184:bool, "Number of POI"=w185:i32)  [unwired: 10 in]
                    n143 = case shown="False" w184 {
                      tunnel: w185 -> [w197 _]
                      frame False {
                        w195 = TRUE
                        w200 = T13."Enabled" ("Disabled")
                        # "Not cancelled. Auto-generate POIs."
                        n144 = global read "gl_ROI Entry UI globals.vi" "ROI entry ctrl refs"() -> (w191:T15)
                        n145 = call "fg_ROI Management.vi"("Function"=ROI_management_FG_states."Clear All") -> ("error out"=w190:errorcluster)  [unwired: 5 in, 5 out]
                        n146 = call "ROI entry-Clear ROI overlay.vi"("error in (no error)"=w190) -> ("Image Out"=w189:T3)  [unwired: 9 in, 1 out]
                        n147 = Unbundle By Name(w191) -> ("Image Display"=w192:refnum<vi>)
                        n148 = call "Auto generate POIs.vi"("Number of POI to generate"=w197, "Image refnum in"=w189) -> ("POI Array"=w198:T21[], "Number of POI generated"=w199:i32)  [unwired: 8 in]
                        n149 = call "ROI entry-Get selected Z-plane index.vi"() -> ("Z-plane selector (index)"=w188:i32)  [unwired: 10 in, 1 out]
                        n150 = global write "gl_ROI Entry UI globals.vi" "Input Mode"(ROI_input_mode."Point-Line-Plane" ("t")) -> ()
                        n151 = Initialize Array(w188, w199) -> (w187:i32[])
                        n152 = property class="ImageControl"(reference=w192, "Line Tool Button Visible"=w195, "Point Tool Button Visible"=w195) -> ()  [unwired: 1 in, 2 out]
                        n153 = call "ROI entry screen-main buttons management.vi"("Acquisition button boolean text"="Functional Acquisition" ("Boolean Text.Text"), "Imaging button disabled?"=T13."Disabled and Grayed Out" ("Disabled"), "Acquisition button disabled?"=w200, "Done button disabled?"=w200) -> ()  [unwired: 8 in]
                        n154 = call "Apply ROIs.vi"("Mode (Redraw All)"=enum16{"Redraw All", "Draw Last"}."Redraw All", "ROIs Info []"=w198, 11:w187) -> ()  [unwired: 5 in, 4 out]
                      }
                      frame True {
                        # "Cancelled"
                      }
                    }
                  }
                }
              }
              frame Enabled {
                n155 = call "POI Gen Engine.vi"("Function"=Duplicate_POI_function_enum."Generate") -> ()  [unwired: 10 in, 1 out]
              }
            }
          }
          event "POI Density": Value Change {
            n156 = event-data() -> ()  [unwired: 1 in, 1 out]
            n157 = global read "General Globals.vi" "First autogen"() -> (w207:bool)
            n158 = case shown="False" w207 {
              frame False {
                n159 = call "POI Gen Engine.vi"("Function"=Duplicate_POI_function_enum."Adjust number of POI") -> ()  [unwired: 10 in, 1 out]
              }
              frame True {
              }
            }
          }
          event "Clear All": Value Change {
            n160 = event-data() -> ()  [unwired: 1 in, 1 out]
            n161 = call "ROI entry-Event handler-Clear All ROI.vi"() -> ()  [unwired: 12 in]
          }
          event "Clear Last": Value Change {
            # "WARNING!\nMore work may be needed"
            n162 = event-data() -> ()  [unwired: 1 in, 1 out]
            n163 = call "ROI entry-Get last ROI ID.vi"() -> ("error out"=w211:errorcluster, "NO ROI"=w210:bool, "ROI ID Enum"=w209:T17)  [unwired: 8 in, 1 out]
            n164 = call "ROI entry-Handle ROI change.vi"("error in (no error)"=w211, "ROI management"=ROI_management_FG_states."Clear Last" ("Function")) -> ("No ROI"=w213:bool, "Number of ROI"=w212:i32)  [unwired: 7 in, 1 out]
            n165 = case shown="False" w213 {
              tunnel: w212 -> [w215 _]
              tunnel: w210 -> [_ w219]
              tunnel: w209 -> [_ w218]
              frame False {
                # "Some ROI exist"
                n166 = local read "Arb Plane Entry"() -> (w216:bool)
                n167 = case shown="True" w216 {
                  tunnel: w215 -> [w217 _]
                  frame True {
                    # "Arb. Plane Entry mode is active"
                    n168 = call "ROI entry screen-Arb plane UI setup.vi"("Number of ROI"=w217) -> ()  [unwired: 11 in]
                  }
                  frame False {
                    # "Arb. Plane Entry mode is not active"
                  }
                }
              }
              frame True {
                # "No ROIs specified"
                n169 = case shown="False" w219 {
                  tunnel: w218 -> [w221 _]
                  frame False {
                    n170 = call "ROI entry-Set ROI tool on Clear All.vi"("Last ROI ID Enum"=w221) -> ()  [unwired: 10 in, 1 out]
                  }
                  frame True {
                  }
                }
                n171 = call "ROI entry-Actions on all ROI cleared.vi"("No ROIs (T)"=TRUE ("empty?")) -> ()  [unwired: 11 in]
              }
            }
          }
          event "POISelect Array": Value Change {
            n172 = event-data() -> ()  [unwired: 1 in, 1 out]
            n173 = disable-structure shown="Disabled" {
              frame Disabled {
                n174 = local read "POISelect Array"() -> (w228:cluster{"System Array":dbl[], "Boolean":bool}[])
                n175 = call "POISelection.vi"("POISelectArrayIn"=w228) -> ("POI array"=w227:dbl[][])  [unwired: 9 in, 1 out]
                n176 = call "ROI entry-Get selected Z-plane index.vi"() -> ("Z-plane selector (index)"=w222:i32)  [unwired: 10 in, 1 out]
                n177 = call "ROI entry-Clear ROI overlay.vi"() -> ("error out"=w225:errorcluster, "Image Out"=w224:T3)  [unwired: 10 in]
                n178 = call "ROI entry-Get Max Proj setting.vi"() -> ("Max Z-projection setting's value"=w223:bool)  [unwired: 10 in, 1 out]
                n179 = for {
                  tunnel: w227 -> [w235] mode=indexing
                  shift-right: [w238] -> w226
                  shift-left: w224 -> [w237]
                  tunnel: w222 -> [w231]
                  tunnel: w225 -> [_]
                  tunnel: w223 -> [w229]
                  n180 = Index Array(array=w235, index=3) -> (element=w233:dbl)
                  n181 = Equal?(x=w233, y=w231) -> (x = y?=w232:bool)
                  n182 = Delete From Array(array=w235, index=0) -> (deleted portion=w230:dbl, array with subset deleted=w236:dbl[])  [unwired: 1 in]
                  n183 = case shown="False" w229 {
                    tunnel: [w244 w255] -> w238
                    tunnel: w237 -> [w243 w254]
                    tunnel: w236 -> [w242 w253]
                    tunnel: w232 -> [w241 _]
                    tunnel: w230 -> [w240 w252]
                    frame False {
                      n184 = case shown="True" w241 {
                        tunnel: [w245 w250] -> w244
                        tunnel: w243 -> [w245 w249]
                        tunnel: w240 -> [_ w248]
                        tunnel: w242 -> [_ w246]
                        frame False {
                        }
                        frame True {
                          n185 = Increment(x=w248) -> (x+1=w247:dbl)
                          n186 = call "PointOverlayV1.vi"("Point"=w246, "Count"=w247, "Image1"=w249) -> ("Image1 Out"=w250:T3)  [unwired: 8 in]
                        }
                      }
                    }
                    frame True {
                      n187 = Increment(x=w252) -> (x+1=w251:dbl)
                      n188 = call "PointOverlayV1.vi"("Point"=w253, "Count"=w251, "Image1"=w254) -> ("Image1 Out"=w255:T3)  [unwired: 8 in]
                    }
                  }
                }
                n189 = call "ROI entry-Image display write.vi"("Value"=w226) -> ()  [unwired: 4 in, 1 out]
              }
              frame Enabled {
              }
            }
          }
          event "Acquisition", "Live Imaging", "Done/Close": Value Change {
            n190 = event-data() -> ("CtlRef"=w258:refnum<vi>)  [unwired: 1 in]
            n191 = call "ROI entry-Event handler-Completion.vi"("Ctrl ref of the control that caused the user event"=w258) -> ("Exit"=w256:bool, "Imaging Mode"=w257:T6)  [unwired: 9 in]
          }
          event "Scan dwell time per pixel (us)", "Trial Length (sec)": Value Change {
            # "Adjusts the Experiment Time and Cool-down time value to the theoretical calculated values which result from the fact that the acquisition time is always an integer multiple of the cycle time."
            n192 = event-data() -> ()  [unwired: 1 in, 1 out]
            n193 = call "Limit entered trial length.vi"() -> ("error out"=w259:errorcluster)  [unwired: 11 in]
            n194 = call "ROI entry screen-Adjust to correct times.vi"("error in (no error)"=w259) -> ()  [unwired: 9 in, 2 out]
          }
          event "Enable funct. stimulus", "Funct stim.trig.delay (sec)": Value Change {
            n195 = event-data() -> ()  [unwired: 1 in, 1 out]
            n196 = flat-sequence {
              frame #0 {
                # "Prevents entering trigger delays <1ms"
                n197 = Greater Or Equal?(x="Funct stim.trig.delay (sec)", y=0.001) -> (x >= y?=w262:bool)
                n198 = Select(t="Funct stim.trig.delay (sec)", s=w262, f=0.0) -> (s? t:f=w261:dbl)
                n199 = local write "Funct stim.trig.delay (sec)"(w261) -> ()
              }
              frame #1 {
                n200 = call "Stimulus trigger delay event handler.vi"() -> ()  [unwired: 12 in]
              }
            }
          }
          event "Cool-down time (s)", "Enable cool-down time": Value Change {
            # "Adjusts the Experiment Time and Cool-down time value to the theoretical calculated values which result from the fact that the acquisition time is always an integer multiple of the cycle time."
            n201 = event-data() -> ()  [unwired: 1 in, 1 out]
            n202 = call "ROI entry screen-Adjust to correct times.vi"() -> ()  [unwired: 10 in, 2 out]
          }
          event "Funct stim.trig.delay (sec)", "Enable funct. stimulus": Mouse Enter {
            # "Stops the \"Stimulus trigger delay\" control blinking if blinking was triggered."
            n203 = event-data() -> ()  [unwired: 1 in, 1 out]
            n204 = call "ROI entry-Stop trig delay blinking.vi"() -> ()  [unwired: 12 in]
          }
          event Panel Close {
            w265 = TRUE ("Stop loop")
            n205 = event-data() -> ()  [unwired: 1 in, 1 out]
          }
        }
      }
      frame True {
        # "Initialisation"
        n206 = flat-sequence {
          tunnel: w267 -> [w306]
          tunnel: [w306] -> w266
          tunnel: w266 -> [w312]
          tunnel: [w313] -> w268
          frame #0 {
            n207 = control-ref of="Image Display"() -> (w289:refnum<vi>)
            n208 = control-ref of="Z-Plane Selector"() -> (w286:refnum<vi>)
            n209 = control-ref of="Done/Close"() -> (w277:refnum<vi>)
            n210 = control-ref of="Live Imaging"() -> (w278:refnum<vi>)
            n211 = control-ref of="Acquisition"() -> (w279:refnum<vi>)
            n212 = control-ref of="Equal size"() -> (w284:refnum<vi>)
            n213 = control-ref of="Arb Plane Entry"() -> (w291:refnum<vi>)
            n214 = control-ref of="Whole plane"() -> (w303:refnum<vi>)
            n215 = control-ref of="Clear Last"() -> (w292:refnum<vi>)
            n216 = control-ref of="Clear All"() -> (w293:refnum<vi>)
            n217 = control-ref of="Max Z Proj"() -> (w299:refnum<vi>)
            n218 = control-ref of="Enable funct. stimulus"() -> (w274:refnum<vi>)
            n219 = control-ref of="Enable cool-down time"() -> (w272:refnum<vi>)
            n220 = control-ref of="POI dwell time (us)"() -> (w280:refnum<vi>)
            n221 = control-ref of="Scan dwell time per pixel (us)"() -> (w281:refnum<vi>)
            n222 = control-ref of="# of planes"() -> (w282:refnum<vi>)
            n223 = control-ref of="Zoom"() -> (w283:refnum<vi>)
            n224 = control-ref of="Number of lines left"() -> (w287:refnum<vi>)
            n225 = control-ref of="Trial Length (sec)"() -> (w294:refnum<vi>)
            n226 = control-ref of="# POI"() -> (w297:refnum<vi>)
            n227 = control-ref of="Zplane ind"() -> (w300:refnum<vi>)
            n228 = control-ref of="Wavelength (nm)"() -> (w302:refnum<vi>)
            n229 = control-ref of="Number of Trials"() -> (w304:refnum<vi>)
            n230 = control-ref of="Funct stim.trig.delay (sec)"() -> (w305:refnum<vi>)
            n231 = control-ref of="Cool-down time (s)"() -> (w273:refnum<vi>)
            n232 = control-ref of="Motor Z ind. (um)"() -> (w271:refnum<vi>)
            n233 = control-ref of="AOL Z ind. (um)"() -> (w270:refnum<vi>)
            n234 = control-ref of="Channel"() -> (w285:refnum<vi>)
            n235 = control-ref of="Palette Type"() -> (w295:refnum<vi>)
            n236 = control-ref of="Line Mode"() -> (w301:refnum<vi>)
            n237 = control-ref of="ROI move mode"() -> (w275:refnum<vi>)
            n238 = control-ref of="Z-stack folder path"() -> (w288:refnum<vi>)
            n239 = control-ref of="POI Density"() -> (w290:refnum<vi>)
            n240 = control-ref of="Intensity slider"() -> (w296:refnum<vi>)
            n241 = control-ref of="Step size (µm)"() -> (w276:refnum<vi>)
            n242 = Bundle By Name(cluster=T15 {"Done button"=refnum, "Imaging button"=refnum, "Acquisition button"=refnum, "POI dwell time (us)"=refnum, "Scan dwell time per pixel (us)"=refnum, "# of planes"=refnum, "Zoom Ctrl"=refnum, "Equal size"=refnum, "Channel"=refnum, "Image Display"=refnum, "Z-Plane Selector"=refnum, "Number of lines left"=refnum, "Z-stack folder path"=refnum, "POI Density"=refnum, "Arb Plane Entry"=refnum, "Whole plane"=refnum, "Clear Last"=refnum, "Clear All"=refnum, "Trial Length (sec)"=refnum, "Palette Type"=refnum, "Intensity slider"=refnum, "# POI"=refnum, "Max Z Proj"=refnum, "Zplane ind"=refnum, "Wavelength (nm)"=refnum, "Number of Trials"=refnum, "Funct stim.trig.enable"=refnum, "Funct stim.trig.delay (s)"=refnum, "Line Mode"=refnum, "Step size (µm)"=refnum, "ROI move mode"=refnum, "Cool-down time (s)"=refnum, "Enable cool-down time"=refnum, "Motor Z ind. (um)"=refnum, "AOL Z ind. (um)"=refnum} ("Ctrl refs cluster"), "Done button"=w277, "Imaging button"=w278, "Acquisition button"=w279, "POI dwell time (us)"=w280, "Scan dwell time per pixel (us)"=w281, "# of planes"=w282, "Zoom Ctrl"=w283, "Equal size"=w284, "Channel"=w285, "Image Display"=w289, "Z-Plane Selector"=w286, "Number of lines left"=w287, "Z-stack folder path"=w288, "POI Density"=w290, "Arb Plane Entry"=w291, "Whole plane"=w303, "Clear Last"=w292, "Clear All"=w293, "Trial Length (sec)"=w294, "Palette Type"=w295, "Intensity slider"=w296, "# POI"=w297, "Max Z Proj"=w299, "Zplane ind"=w300, "Line Mode"=w301, "Wavelength (nm)"=w302, "Number of Trials"=w304, "Funct stim.trig.enable"=w274, "Funct stim.trig.delay (s)"=w305, "Step size (µm)"=w276, "ROI move mode"=w275, "Cool-down time (s)"=w273, "Enable cool-down time"=w272, "Motor Z ind. (um)"=w271, "AOL Z ind. (um)"=w270) -> (w298:T15)
            n243 = global write "gl_ROI Entry UI globals.vi" "ROI entry ctrl refs"(w298) -> ()
          }
          frame #1 {
            n244 = control-ref of="Pane"() -> (w311:refnum<vi>)
            n245 = control-ref of="Pane 2"() -> (w310:refnum<vi>)
            n246 = Build Array(w311, w310) -> (w309:refnum<vi>[])
            n247 = call "ROI entry-Initialisation.vi"("Pane refs array"=w309, "User Events Cluster"=w312) -> ("Open file dialogue window"=w313:bool)  [unwired: 9 in]
            n248 = call "fgv_Enforce AOL Z repeat.vi"("Function"=Read_Write_Enum."Write", "Enforce AOL Z repeat"=FALSE) -> ()  [unwired: 8 in, 2 out]
          }
        }
      }
    }
  }
  n249 = call "ROI entry-Exit actions.vi"("Imaging Mode"=w8, "Stop loop"=w9, "User Events cluster"=w1) -> ("error out"=w7:errorcluster)  [unwired: 8 in]
  n250 = case shown="False" w9 {
    tunnel: w8 -> [w314 _]
    frame False {
      "Next State" <- w314
    }
    frame True {
    }
  }
  n251 = flat-sequence {
    tunnel: w7 -> [_]
    frame #0 {
      n252 = call "Enable-Disable UI by Z stack.vi"() -> ("Controls refs to enable/disable"=w317:refnum<vi>[])  [unwired: 11 in]
      n253 = call "Enable-Disable UI by Motor Z stack.vi"() -> ("Controls to disable"=w315:refnum<vi>[])  [unwired: 11 in]
      n254 = Request Deallocation(TRUE ("flag")) -> ()
      n255 = local write "Done/Close"(FALSE ("Done/Close")) -> ()
      n256 = Build Array (concatenate)(w317, w315) -> (w316:refnum<vi>[])
      n257 = call "Enable-Disable Encoder UI conditionally.vi"() -> ()  [unwired: 11 in, 1 out]
      n258 = call "Enable-Disable UI Elements.vi"("Enable/Disable"=T13."Enabled", "Ctrl ref's"=w316) -> ()  [unwired: 9 in, 1 out]
    }
  }
